vi "Set Solenid.vi"(8 "On":bool, 9 "Off":bool, 11 "Solenid Ref.":string="My Solenoid RefNum") -> ()   [LabVIEW 2015, in "hhVI.lvlib"]
uses:
  <vilib>/Rock Robotics/WPI/Solenoid/WPI_SolenoidValue.ctl
  <vilib>/Rock Robotics/WPI/Solenoid/WPI_SolenoidSetEnum.vi
  hhVI.lvlib
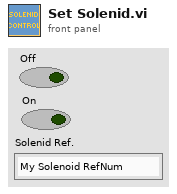
[diagram p1: front panel]
types:
  T1 = typedef "WPI_SolenoidDevRef.ctl" = cluster{"DevStatus":errorcluster, "Pneumatics Control Module":u8, "Forward Solenoid Channel":T2, "Reverse Solenoid Channel":T2}
  T2 = typedef "WPI_SolenoidChannel.ctl" = enum8{"Solenoid 0", "Solenoid 1", "Solenoid 2", "Solenoid 3", "Solenoid 4", "Solenoid 5", "Solenoid 6", "Solenoid 7", "Invalid"}
  T3 = typedef "WPI_SolenoidValue.ctl" = enum16{"Off", "On", "Forward", "Reverse"}
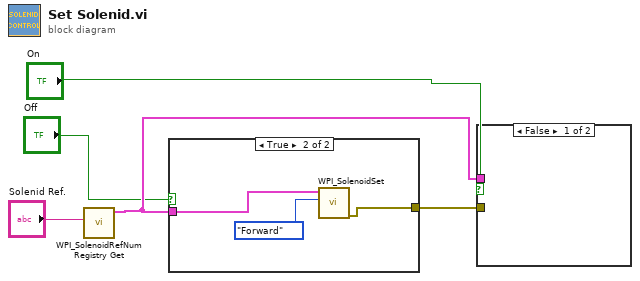
[diagram p0: block diagram]
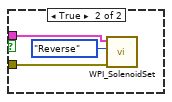
[diagram p2: hidden frame]
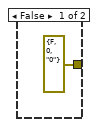
[diagram p3: hidden frame]
diagram:
  n1 = call <vilib>:"WPI_SolenoidRefNum Registry Get.vi"("refnum name"="Solenid Ref.") -> ("SolenoidDevRef"=w4:T1)  [unwired: 9 in, 1 out]
  n2 = case shown="True" "Off" {
    tunnel: w4 -> [_ w7]
    tunnel: [errorcluster {"status"=FALSE, "code"=0, "source"="0"} ("error out") w8] -> w5
    frame False {
    }
    frame True {
      n3 = call-poly <vilib>:"WPI_SolenoidSet.vi"("Value"=WPI_SolenoidValue."Forward", "SolenoidDevRef"=w7) -> ("error out"=w8:errorcluster)  [unwired: 8 in, 1 out]
    }
  }
  n4 = case shown="False" "On" {
    tunnel: w4 -> [_ w12]
    tunnel: w5 -> [_ w11]
    frame False {
    }
    frame True {
      n5 = call-poly <vilib>:"WPI_SolenoidSet.vi"("error in (no error)"=w11, "Value"=WPI_SolenoidValue."Reverse", "SolenoidDevRef"=w12) -> ()  [unwired: 7 in, 2 out]
    }
  }
